vi "Auto Locate.vi"(2 "Aim?":bool, 3 "Autonomous?":bool) -> (0 "X Drive Arcade":dbl, 1 "Set?":bool)   [LabVIEW 2012]
uses:
  BotStatus.vi
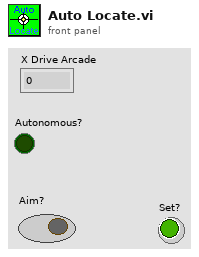
[diagram p1: front panel]
types:
  T1 = cluster{"Target Position X":dbl, "Target Position Y":dbl, "Target Found":bool}
  T2 = typedef "WPI_ServoDeviceRef.ctl" = cluster{"DeviceStatus":errorcluster, "Digital Module":T3, "PWM Channel":T4, "DeadBand":T5}
  T3 = typedef "FPGA_TypedefDigitalModule.ctl" = enum16{"Digital Module 1", "Digital Module 2"}
  T4 = typedef "FPGA_DIOPWMChannel.ctl" = enum8{"PWM 1", "PWM 2", "PWM 3", "PWM 4", "PWM 5", "PWM 6", "PWM 7", "PWM 8", "PWM 9", "PWM 10", "Invalid"}
  T5 = typedef "WPI_PWMDeadband.ctl" = cluster{"Name":string, "maxPositivePwm":i32, "minPositivePwm":i32, "centerPwm":i32, "maxNegativePwm":i32, "minNegativePwm":i32, "angularRange":u16}
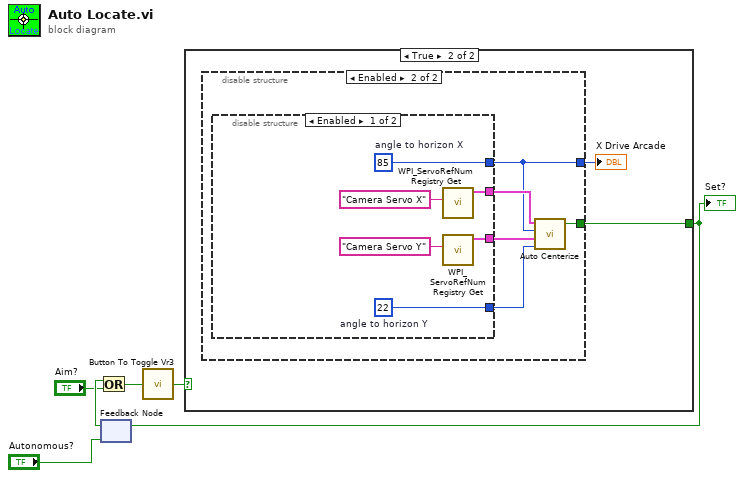
[diagram p0: block diagram]
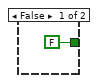
[diagram p2: hidden frame]
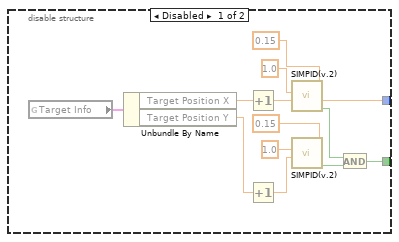
[diagram p3: hidden frame]
diagram:
  n1 = feedback #1("Autonomous?") -> (w4:bool)
  n2 = Or(x=w4, y="Aim?") -> (x .or. y?=w5:bool)
  n3 = call "Button To Toggle Vr3.vi"("InValue"=w5) -> ("Result"=w6:bool)
  n4 = case shown="True" w6 {
    tunnel: [FALSE w9] -> w1
    frame False {
    }
    frame True {
      n5 = disable-structure shown="Enabled" {
        disable-tunnel: [w12 w25] -> w9
        disable-tunnel: [w11 w24] -> w8
        frame Disabled {
          n6 = global read "BotStatus.vi" "Target Info"() -> (w23:T1)
          n7 = Unbundle By Name(w23) -> ("Target Position X"=w18:dbl, "Target Position Y"=w22:dbl)
          n8 = Increment(x=w18) -> (x+1=w17:dbl)
          n9 = Increment(x=w22) -> (x+1=w21:dbl)
          n10 = call "SIMPID(v.2).vi"("Range"=0.15, "Current Point"=w17, "Set Point"=1.0) -> ("On Target"=w13:bool, "result"=w11:dbl)  [unwired: 7 in]
          n11 = call "SIMPID(v.2).vi"("Range"=0.15, "Current Point"=w21, "Set Point"=1.0) -> ("On Target"=w14:bool, "result"=w10:dbl)  [unwired: 7 in]
          n12 = And(x=w13, y=w14) -> (x .and. y?=w12:bool)
        }
        frame Enabled {
          n13 = disable-structure shown="Enabled" {
            disable-tunnel: [w33 _] -> w28
            disable-tunnel: [w31 _] -> w27
            disable-tunnel: [w30 _] -> w24
            disable-tunnel: [w29 _] -> w26
            frame Enabled {
              w29 = u16 22  # angle to horizon Y
              w30 = u16 85  # angle to horizon X
              n14 = call <vilib>:"WPI_ServoRefNum Registry Get.vi"("refnum name"="Camera Servo X") -> ("ServoDeviceRef"=w33:T2)  [unwired: 9 in, 1 out]
              n15 = call <vilib>:"WPI_ServoRefNum Registry Get.vi"("refnum name"="Camera Servo Y") -> ("ServoDeviceRef"=w31:T2)  [unwired: 9 in, 1 out]
            }
            frame Disabled {
            }
          }
          n16 = call "Auto Centerize.vi"("angle to horizon Y"=w26, "Camera Y ServoDeviceRef"=w27, "angle to horizon X"=w24, "Camera X ServoDeviceRef"=w28) -> ("Centerized?"=w25:bool)  [unwired: 1 in, 1 out]
        }
      }
      "X Drive Arcade" <- w8
    }
  }
  "Set?" <- w1
  n17 = feedback-in #1(w1) -> ()
